vi "Set Log File Description.vi"(6 "timeout (ms)":i32=-1, 8 "error in (no error)":errorcluster, 10 "log_file_description":string, 11 "FlexLogger_gRPC in":refnum<class "FlexLogger_gRPC.lvclass">) -> (0 "error out":errorcluster, 3 "FlexLogger_gRPC out":refnum<class "FlexLogger_gRPC.lvclass">)   [LabVIEW 2020, in "FlexLogger_gRPC.lvlib" / "FlexLogger_gRPC.lvclass"]
doc: "Set the Log File description of the Current project"
uses:
  FlexLogger_gRPC.lvclass
  FlexLogger_client/RPC Messages/flexlogger_SetLogFileDescriptionRequest.ctl
  FlexLogger_client/RPC Messages/flexlogger_ElementIdentifier.ctl
  FlexLogger_gRPC.lvclass/FlexLogger_gRPC.ctl
  FlexLogger_client/FlexLogger_client.lvlib
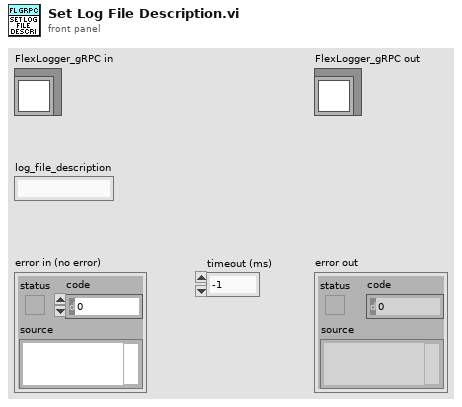
[diagram p1: front panel]
types:
  T1 = typedef "FlexLogger_client.lvlib/flexlogger_SetLogFileDescriptionRequest.ctl" = cluster{"document_identifier":T2, "log_file_description":string}
  T2 = typedef "FlexLogger_client.lvlib/flexlogger_ElementIdentifier.ctl" = cluster{"project_id":string, "file_name":string, "element_id":string, "subpart_id":string}
  T3 = typedef "grpc-lvsupport-release.lvlib/grpcId.ctl" = u64
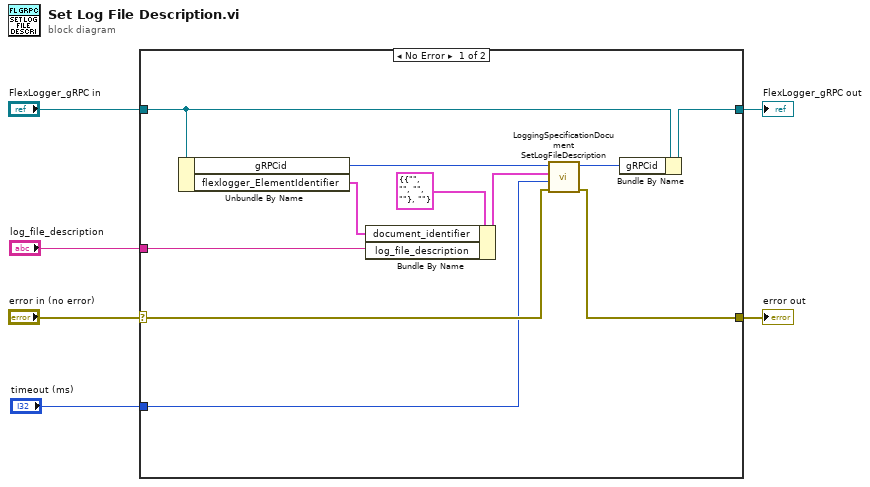
[diagram p0: block diagram]
diagram:
  n1 = case shown="No Error" "error in (no error)" {
    selector: "error in (no error)" -> [w13 w18]
    tunnel: "FlexLogger_gRPC in" -> [w17 w19]
    tunnel: [w16 w19] -> w6
    tunnel: [w12 w18] -> w4
    tunnel: "timeout (ms)" -> [w11 _]
    tunnel: "log_file_description" -> [w7 _]
    frame No Error {
      n2 = Unbundle By Name(w17) -> ("gRPCid"=w15:T3, "flexlogger_ElementIdentifier"=w9:T2)
      n3 = Bundle By Name(cluster=T1 {"document_identifier"={"project_id"="", "file_name"="", "element_id"="", "subpart_id"=""}, "log_file_description"=""} ("Request Data"), "document_identifier"=w9, "log_file_description"=w7) -> (w8:T1)
      n4 = call "LoggingSpecificationDocument SetLogFileDescription.vi"("error in"=w13, "timeout (ms)"=w11, "Request Data"=w8, "gRPC ID"=w15) -> ("error out"=w12:errorcluster, "gRPC ID out"=w14:T3)  [unwired: 5 in, 1 out]
      n5 = Bundle By Name(cluster=w17, "gRPCid"=w14) -> (w16:refnum<class "FlexLogger_gRPC.lvclass">)
    }
    frame Error {
    }
  }
  "error out" <- w4
  "FlexLogger_gRPC out" <- w6
